vi "Creat bounding sphere.vi"(1 "Triangles":T2[](array[typedef])) -> (0 "Bounding sphere":T1)   [LabVIEW 2014]
uses:
  Typedefs/Triangle.ctl
  Typedefs/Sphere.ctl
panel:
  # "PN 13/03/2015"
  # "Vertices"
  # "Edges"
  # "Unit normal"
  # "Edge unit normals"
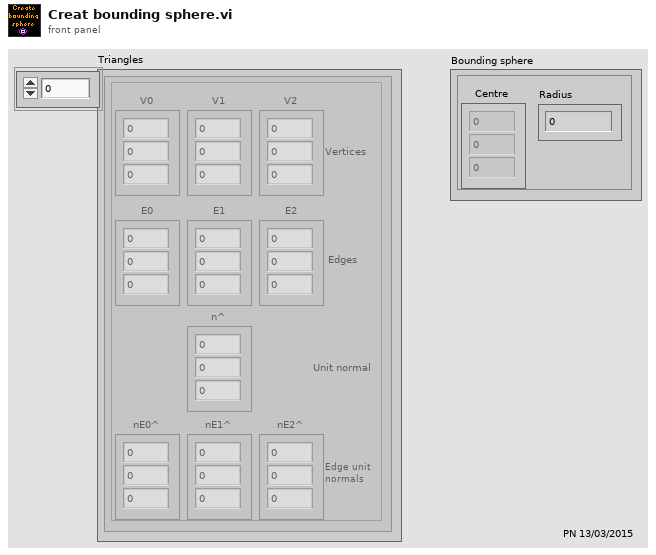
[diagram p1: front panel]
types:
  T1 = typedef "Sphere.ctl" = cluster{"Centre":sgl[], "Radius":sgl}
  T2 = typedef "Triangle.ctl" = cluster{"V0":sgl[], "V1":sgl[], "V2":sgl[], "E0":sgl[], "E1":sgl[], "E2":sgl[], "n^":sgl[], "nE0^":sgl[], "nE1^":sgl[], "nE2^":sgl[]}
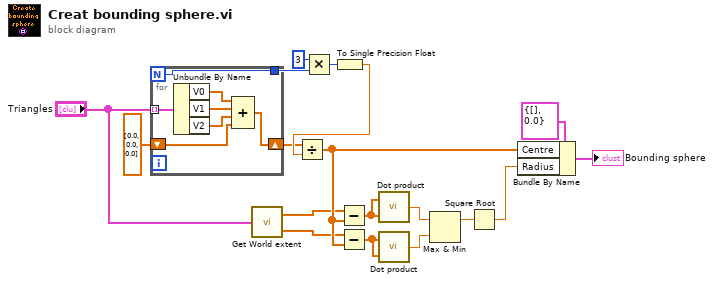
[diagram p0: block diagram]
diagram:
  n1 = for {
    N -> [w20]
    tunnel: "Triangles" -> [w25] mode=indexing
    shift-right: [w21] -> w12
    shift-left: sgl[] [0.0, 0.0, 0.0] -> [w19]
    tunnel: [w20] -> w17
    n2 = Unbundle By Name(w25) -> ("V0"=w24:sgl[], "V1"=w22:sgl[], "V2"=w23:sgl[])
    n3 = Compound Arithmetic op=ADD(w24, w22, w23, w19) -> (w21:sgl[])
  }
  n4 = call "Get World extent.vi"("Triangles"="Triangles") -> ("Pmax (x, y, z)"=w2:sgl[], "Pmin (x, y, z)"=w1:sgl[])
  n5 = Multiply(x=3, y=w17) -> (x*y=w15:i32)
  n6 = To Single Precision Float(number=w15) -> (single precision float=w14:sgl)
  n7 = Divide(x=w12, y=w14) -> (x/y=w3:sgl[])
  n8 = Subtract(x=w2, y=w3) -> (x-y=w10:sgl[])
  n9 = Subtract(x=w1, y=w3) -> (x-y=w9:sgl[])
  n10 = call "Dot product.vi"("B"=w10, "A"=w10) -> ("A . B"=w8:sgl)
  n11 = call "Dot product.vi"("B"=w9, "A"=w9) -> ("A . B"=w7:sgl)
  n12 = Max & Min(x=w8, y=w7) -> (max(x,y)=w6:sgl)  [unwired: 1 out]
  n13 = Square Root(x=w6) -> (sqrt(x)=w5:sgl)
  n14 = Bundle By Name(cluster=T1 {"Centre"=[], "Radius"=0.0} ("Sphere"), "Centre"=w3, "Radius"=w5) -> (→"Bounding sphere":T1)
